vi "test I8.vi"(11 "Test Case In":refnum<class "Build Sequence Test.lvclass">) -> (0 "error out":errorcluster, 3 "Test Case Out":refnum<class "Build Sequence Test.lvclass">)   [LabVIEW 2024, in "Build Sequence Test.lvclass"]
uses:
  Build Sequence Test.lvclass
  C:/Program Files/National Instruments/LabVIEW 2024/vi.lib/Astemes/LUnit/Test Case.lvclass
  <vilib>/Astemes/LUnit/Test Case.lvclass/Test Case.ctl
  4993e8ee-a06a-463a-9684-69129f64d5ce.vi
  <vilib>/Astemes/LUnit/Append Pass Result.vi
  <vilib>/Astemes/LUnit/Append Fail Result.vi
  <vilib>/Astemes/LUnit/Describe Comparison.vi
  4993e8ee-a06a-463a-9684-69129f64d5ce.vi/9c5d11cd-9439-4240-a1ee-d9baace9c924.vi
  <vilib>/Astemes/LUnit/Run In UI.vi
  <vilib>/Utility/error.llb/Clear Errors.vi
  <vilib>/Astemes/LUnit/Describe Variant.vi
  CANopen/CANopen.lvclass
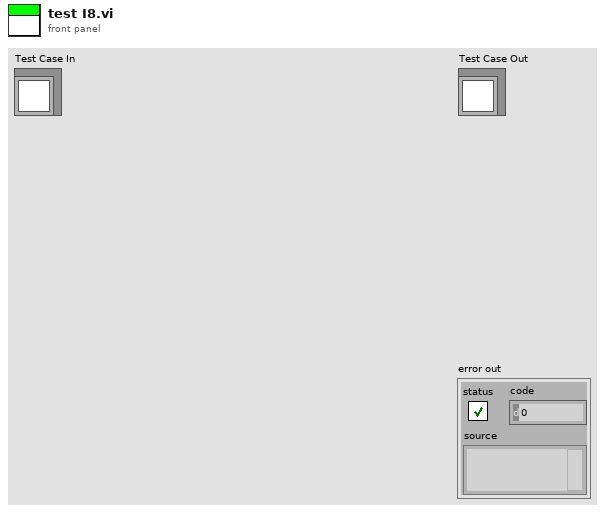
[diagram p1: front panel]
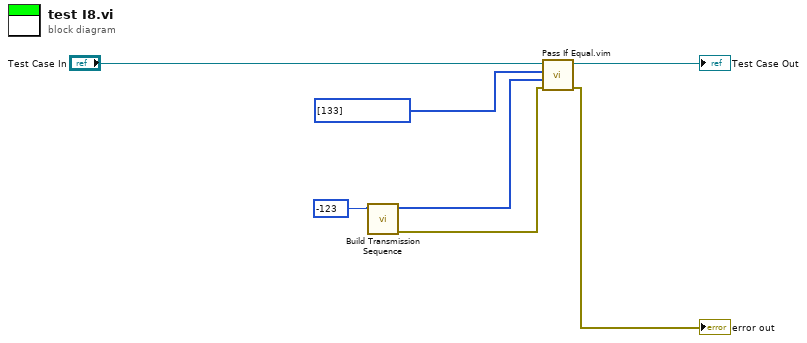
[diagram p0: block diagram]
diagram:
  n1 = call "Build Transmission Sequence.vi"("Data"=i8 -123 ("Numeric")) -> ("error out"=w1:errorcluster, "Transmission Sequence"=w2:u8[])  [unwired: 9 in]
  n2 = call "Pass If Equal.vim"("error in (no error)"=w1, "Actual"=w2, "Expected"=u8[] [133] ("appended array"), "LUnit Test Case In"="Test Case In") -> ("error out"=→"error out":errorcluster, "LUnit Test Case Out"=→"Test Case Out":refnum<class "Build Sequence Test.lvclass">)  [unwired: 6 in]
